vi "Drop Marker.vi"(8 "error in (no error)":errorcluster, 10 "Position":T1, 11 "Maze in":refnum<class "Maze.lvclass">) -> (0 "error out":errorcluster, 3 "Maze out":refnum<class "Maze.lvclass">)   [LabVIEW 2020, in "Maze.lvlib" / "Maze.lvclass"]
uses:
  Maze.lvclass
  Position.ctl
  Maze.lvclass/Maze.ctl
  Maze.lvlib
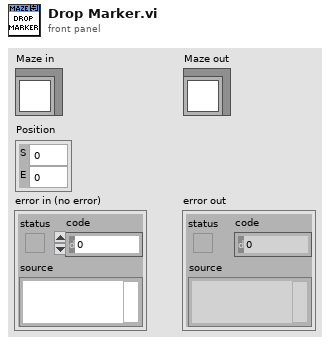
[diagram p1: front panel]
types:
  T1 = typedef "Maze.lvlib/Position.ctl" = cluster{"S":i32, "E":i32}
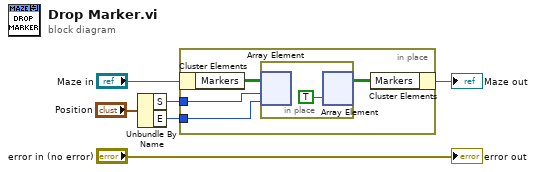
[diagram p0: block diagram]
diagram:
  n1 = Unbundle By Name("Position") -> ("S"=w3:i32, "E"=w2:i32)
  n2 = in-place {
    in-place-border: w3 -> [w8]
    in-place-border: w2 -> [w9]
    n3 = in-place-cluster #1("Maze in") -> ("Markers"=w10:bool[][])
    n4 = in-place {
      n5 = in-place-array #2(w10, w8, w9) -> ()  [unwired: 1 out]
      n6 = in-place-array #2(TRUE ("element")) -> (w7:bool[][])  [unwired: 2 out]
    }
    n7 = in-place-cluster #1("Markers"=w7) -> (→"Maze out":refnum<class "Maze.lvclass">)
  }
  "error out" <- "error in (no error)"
